vi "CreateExportedFunctionVIs.vi"   [LabVIEW 2020]
uses:
  <vilib>/Utility/traverseref.llb/TRef TravTarget.ctl
  6dd5ec1a-3140-4c59-8976-e265b4825e4e.vi
  c28e3e03-bc47-4083-b8a7-f1b137712541.vi
  82b46e61-a036-43bd-a8d9-afcc1ab177d3.vi
  337b4f8b-581d-4fd9-b696-00d79b3d5e3a.vi
  67cb83f1-d3a9-42e9-95c3-879ee97d33c6.vi
  533b81a4-3358-4744-80f6-d38457af82e6.vi
  g_industrial_cam/Camera/Get Pixel Format.vi
  g_industrial_cam/Camera/Set Pixel Format.vi
  g_industrial_cam/Camera/Get Exposure Time Bounds.vi
  g_industrial_cam/Camera/Available Pixel Formats.vi
  g_industrial_cam/Camera/Is Gain Available.vi
  g_industrial_cam/Camera/Get Height Increment.vi
  <vilib>/Comparison/Equal/Equal Functor/Equal Functor.lvclass
  <vilib>/Utility/traverseref.llb/VI Scripting - Traverse.lvlib
  g_industrial_cam/Camera/Camera.lvclass
types:
  T1 = typedef "TRef TravTarget.ctl" = enum16{"FP", "BD", "Other"}
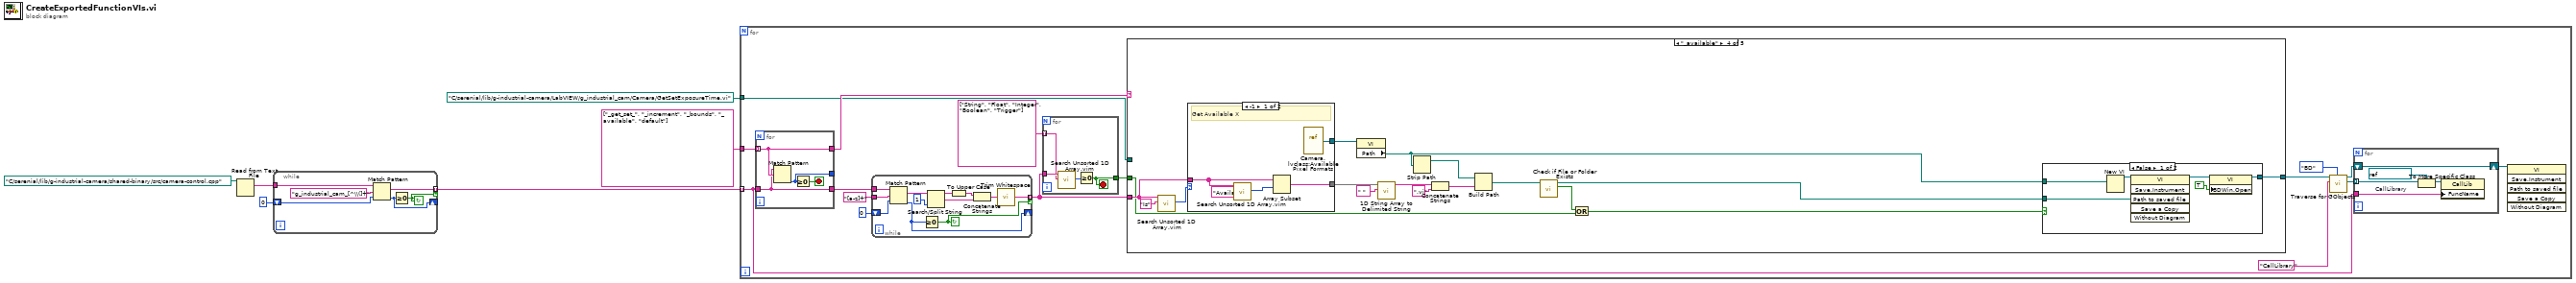
[diagram p0: block diagram]
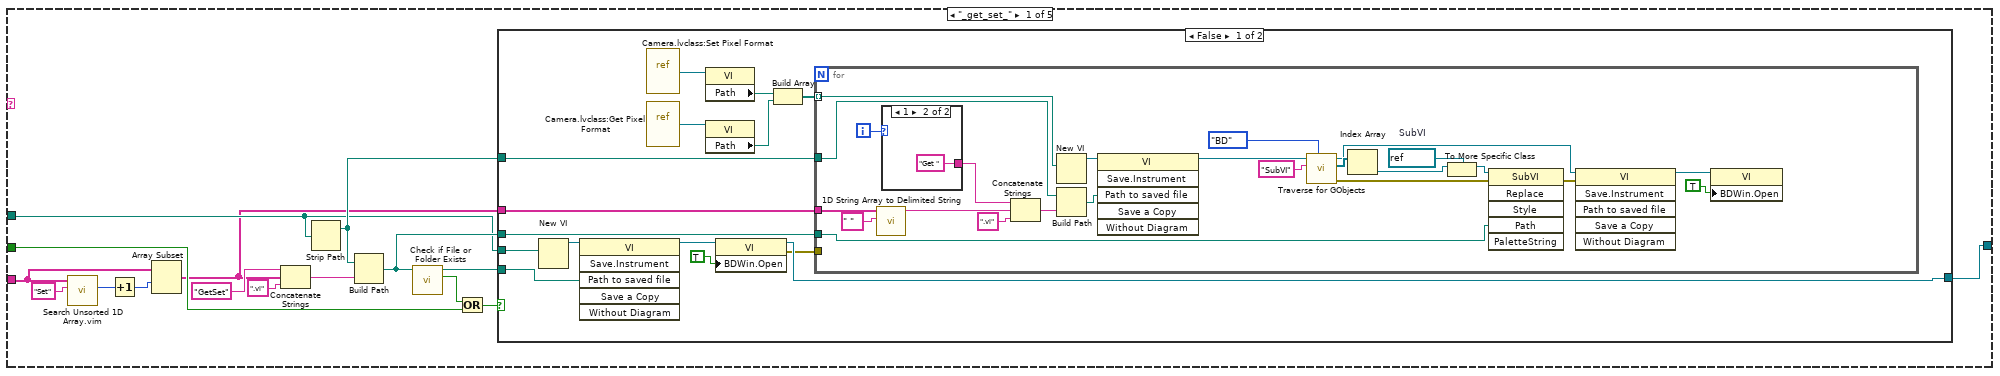
[diagram p2: hidden frame]
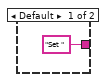
[diagram p3: hidden frame]
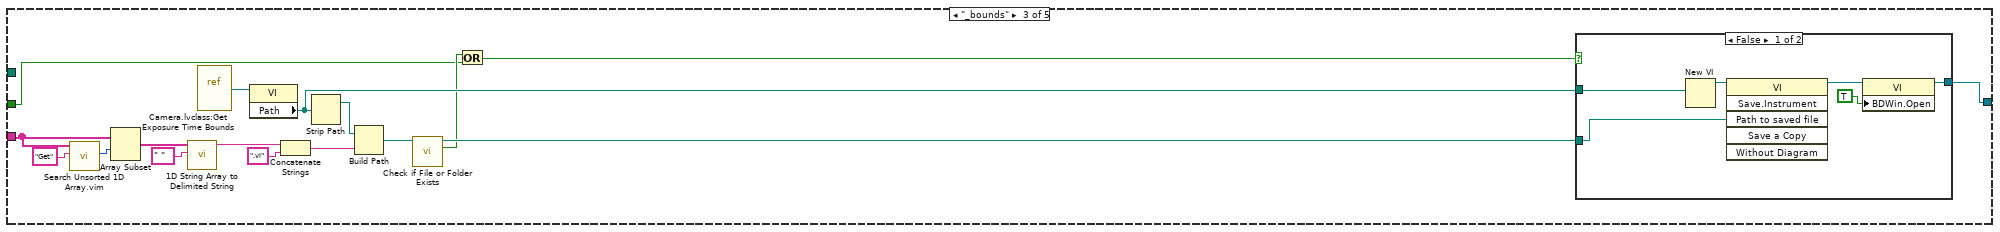
[diagram p6: hidden frame]
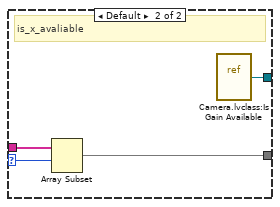
[diagram p8: hidden frame]
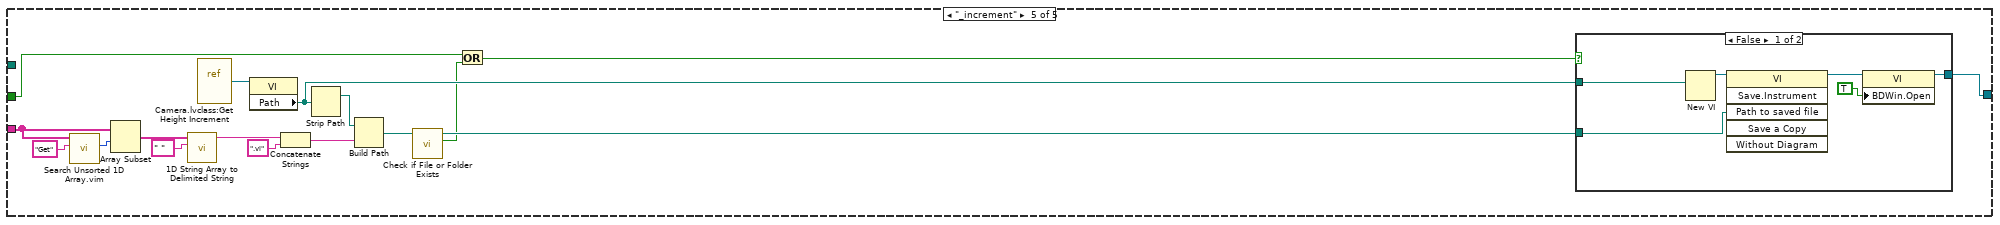
[diagram p10: hidden frame]
diagram:
  n1 = Read from Text File(file (use dialog)=path "C:/serenial/lib/g-industrial-camera/shared-binary/src/camera-control.cpp") -> (text=w1:string)  [unwired: 3 in, 3 out]
  n2 = while {
    tunnel: w1 -> [w12]
    shift-right: [w8] -> _
    shift-left: 0 ("offset (0)") -> [w10]
    tunnel: [w9] -> w5 mode=indexing if=w7
    stop <- w7 continue-if-true
    n3 = Match Pattern(string=w12, regular expression="g_industrial_cam_[^\\(]+", offset (0)=w10) -> (match substring=w9:string, offset past match=w8:i32)  [unwired: 2 out]
    n4 = Greater Or Equal To 0?(x=w8) -> (x >= 0?=w7:bool)
  }
  n5 = for {
    tunnel: w5 -> [w17] mode=indexing
    tunnel: string[] ["_get_set_", "_increment", "_bounds", "_available", "default"] -> [w28]
    tunnel: path "C:/serenial/lib/g-industrial-camera/LabVIEW/g_industrial_cam/Camera/GetSetExposureTime.vi" ("template") -> [w16]
    n6 = for {
      tunnel: w17 -> [w186]
      tunnel: w28 -> [w187] mode=indexing
      tunnel: [w187] -> w27
      tunnel: [w186] -> w26
      tunnel: [w185] -> _
      stop <- w188 stop-if-true
      n7 = Match Pattern(string=w186, regular expression=w187) -> (offset past match=w185:i32)  [unwired: 1 in, 3 out]
      n8 = Greater Or Equal To 0?(x=w185) -> (x >= 0?=w188:bool)
    }
    n9 = while {
      tunnel: w26 -> [w49]
      tunnel: "[a-z]+" ("regular expression") -> [w48]
      shift-right: [w46] -> _
      shift-left: 0 ("offset (0)") -> [w47]
      tunnel: [w38] -> w14 mode=indexing if=w45
      stop <- w45 continue-if-true
      n10 = Match Pattern(string=w49, regular expression=w48, offset (0)=w47) -> (match substring=w43:string, offset past match=w46:i32)  [unwired: 2 out]
      n11 = Greater Or Equal To 0?(x=w46) -> (x >= 0?=w45:bool)
      n12 = Search/Split String(string=w43, offset (0)=1) -> (substring before match=w42:string, match + rest of string=w40:string)  [unwired: 1 in, 1 out]
      n13 = To Upper Case(1:w42) -> (0:w41:string)
      n14 = Concatenate Strings(w41, w40) -> (w39:string)
      n15 = call <vilib>:"Trim Whitespace.vi"("string"=w39) -> ("trimmed string"=w38:string)  [unwired: 1 in]
    }
    n16 = for {
      tunnel: string[] ["String", "Float", "Integer", "Boolean", "Trigger"] -> [w31] mode=indexing
      tunnel: w14 -> [w32]
      tunnel: [w29] -> w13
      stop <- w29 stop-if-true
      n17 = call "Search Unsorted 1D Array.vim"("element"=w31, "unsorted 1D array"=w32) -> ("index of element"=w30:i32)  [unwired: 9 in]
      n18 = Greater Or Equal To 0?(x=w30) -> (x >= 0?=w29:bool)
    }
    n19 = case shown="\"_available\"" w27 {
      tunnel: w14 -> [w57 _ w122 w145 w177]
      tunnel: [w63 _ w111 w134 w166] -> w20
      tunnel: w16 -> [w55 _ _ _ _]
      tunnel: w13 -> [w51 _ w107 w130 w162]
      frame "_get_set_" {
        n20 = call "Search Unsorted 1D Array.vim"("element"="Set", "unsorted 1D array"=w57) -> ("index of element"=w58:i32)  [unwired: 9 in]
        n21 = Increment(x=w58) -> (x+1=w56:i32)
        n22 = Array Subset(array=w57, index=w56) -> (w50:string[])  [unwired: 1 in]
        n23 = Concatenate Strings("GetSet" ("string"), w50, ".vi" ("string")) -> (w64:string)
        n24 = Strip Path(path=w55) -> (stripped path=w62:path)  [unwired: 1 out]
        n25 = Build Path(base path=w62, name or relative path=w64) -> (appended path=w61:path)
        n26 = call <vilib>:"Check if File or Folder Exists.vi"("path"=w61) -> ("file or folder exists?"=w53:bool, "dup path"=w54:path)  [unwired: 8 in, 1 out]
        n27 = Or(x=w53, y=w51) -> (x .or. y?=w52:bool)
        n28 = case shown="False" w52 {
          tunnel: [w80 _] -> w63
          tunnel: w62 -> [w74 _]
          tunnel: w61 -> [w73 _]
          tunnel: w50 -> [w68 _]
          tunnel: w55 -> [w67 _]
          tunnel: w54 -> [w66 _]
          frame False {
            n29 = New VI(10:w67) -> (3:w71:refnum<vi>)  [unwired: 6 in, 1 out]
            n30 = invoke class="VI" method="Save.Instrument"(reference=w71, "Path to saved file"=w66) -> (reference out=w70:refnum<vi>)  [unwired: 4 in, 5 out]
            n31 = vi-ref "Camera.lvclass:Set Pixel Format.vi"() -> (w78:refnum<vi>)
            n32 = vi-ref "Camera.lvclass:Get Pixel Format.vi"() -> (w79:refnum<vi>)
            n33 = property class="VI"(reference=w78) -> ("Path"=w76:path)  [unwired: 1 in, 2 out]
            n34 = property class="VI"(reference=w79) -> ("Path"=w77:path)  [unwired: 1 in, 2 out]
            n35 = property class="VI"(reference=w70, "BDWin.Open"=TRUE ("Block Diagram Window:Open")) -> (reference out=w80:refnum<vi>, error out=w72:errorcluster)  [unwired: 1 in]
            n36 = Build Array(w76, w77) -> (w75:path[])
            n37 = for {
              tunnel: w75 -> [w99] mode=indexing
              tunnel: w74 -> [w100]
              tunnel: w68 -> [w97]
              tunnel: w73 -> [w98]
              tunnel: w72 -> [_]
              i -> [w96]
              w87 = refnum<vi> refnum  # SubVI
              n38 = call <vilib>:"1D String Array to Delimited String.vi"("delimiter"=" ", "string array"=w97) -> ("delimited string"=w103:string)  [unwired: 9 in]
              n39 = case shown="1" w96 {
                tunnel: ["Set " "Get "] -> w95
                frame Default {
                }
                frame 1 {
                }
              }
              n40 = Concatenate Strings(w95, w103, ".vi" ("string")) -> (w101:string)
              n41 = New VI(10:w99) -> (3:w94:refnum<vi>)  [unwired: 6 in, 1 out]
              n42 = Build Path(base path=w100, name or relative path=w101) -> (appended path=w93:path)
              n43 = invoke class="VI" method="Save.Instrument"(reference=w94, "Path to saved file"=w93) -> (reference out=w92:refnum<vi>)  [unwired: 4 in, 5 out]
              n44 = call <vilib>:"Traverse for GObjects.vi"("Traverse Target"=TRef_TravTarget."BD", "Class Name"="SubVI", "VI Refnum"=w92) -> ("error out"=w85:errorcluster, "References"=w89:refnum<vi>[], "dup VI Refnum"=w84:refnum<vi>)  [unwired: 5 in, 1 out]
              n45 = Index Array(array=w89) -> (element=w88:refnum<vi>)  [unwired: 1 in]
              n46 = To More Specific Class(target class=w87, reference=w88) -> (specific class reference=w86:refnum<vi>)  [unwired: 1 in, 1 out]
              n47 = invoke class="SubVI" method="Replace"(reference=w86, error in=w85, "Path"=w98) -> (error out=w83:errorcluster)  [unwired: 3 in, 5 out]
              n48 = invoke class="VI" method="Save.Instrument"(reference=w84, error in=w83) -> (reference out=w82:refnum<vi>)  [unwired: 4 in, 5 out]
              n49 = property class="VI"(reference=w82, "BDWin.Open"=TRUE ("Block Diagram Window:Open")) -> ()  [unwired: 1 in, 2 out]
            }
          }
          frame True {
          }
        }
      }
      frame Default {
      }
      frame "_bounds" {
        n50 = call "Search Unsorted 1D Array.vim"("element"="Get", "unsorted 1D array"=w122) -> ("index of element"=w121:i32)  [unwired: 9 in]
        n51 = Array Subset(array=w122, index=w121) -> (w118:string[])  [unwired: 1 in]
        n52 = call <vilib>:"1D String Array to Delimited String.vi"("delimiter"=" ", "string array"=w118) -> ("delimited string"=w116:string)  [unwired: 9 in]
        n53 = vi-ref "Camera.lvclass:Get Exposure Time Bounds.vi"() -> (w120:refnum<vi>)
        n54 = property class="VI"(reference=w120) -> ("Path"=w115:path)  [unwired: 1 in, 2 out]
        n55 = Concatenate Strings(w116, ".vi" ("string")) -> (w113:string)
        n56 = Strip Path(path=w115) -> (stripped path=w114:path)  [unwired: 1 out]
        n57 = Build Path(base path=w114, name or relative path=w113) -> (appended path=w112:path)
        n58 = call <vilib>:"Check if File or Folder Exists.vi"("path"=w112) -> ("file or folder exists?"=w109:bool, "dup path"=w110:path)  [unwired: 8 in, 1 out]
        n59 = Or(x=w109, y=w107) -> (x .or. y?=w108:bool)
        n60 = case shown="False" w108 {
          tunnel: w115 -> [w128 _]
          tunnel: [w125 _] -> w111
          tunnel: w110 -> [w124 _]
          frame False {
            n61 = New VI(10:w128) -> (3:w129:refnum<vi>)  [unwired: 6 in, 1 out]
            n62 = invoke class="VI" method="Save.Instrument"(reference=w129, "Path to saved file"=w124) -> (reference out=w127:refnum<vi>)  [unwired: 4 in, 5 out]
            n63 = property class="VI"(reference=w127, "BDWin.Open"=TRUE ("Block Diagram Window:Open")) -> (reference out=w125:refnum<vi>)  [unwired: 1 in, 1 out]
          }
          frame True {
          }
        }
      }
      frame "_available" {
        n64 = call "Search Unsorted 1D Array.vim"("element"="Is", "unsorted 1D array"=w145) -> ("index of element"=w144:i32)  [unwired: 9 in]
        n65 = case shown="-1" w144 {
          selector: w144 -> [_ w154]
          tunnel: w145 -> [w150 w155]
          tunnel: [w147 w153] -> w143
          tunnel: [w148 w152] -> w141
          frame -1 {
            # "Get Available X"
            n66 = call "Search Unsorted 1D Array.vim"("element"="Available", "unsorted 1D array"=w150) -> ("index of element"=w149:i32)  [unwired: 9 in]
            n67 = Array Subset(array=w150, index=w149) -> (w148:string[])  [unwired: 1 in]
            n68 = vi-ref "Camera.lvclass:Available Pixel Formats.vi"() -> (w147:refnum<vi>)
          }
          frame Default {
            # "is_x_avaliable"
            n69 = Array Subset(array=w155, index=w154) -> (w152:string[])  [unwired: 1 in]
            n70 = vi-ref "Camera.lvclass:Is Gain Available.vi"() -> (w153:refnum<vi>)
          }
        }
        n71 = property class="VI"(reference=w143) -> ("Path"=w138:path)  [unwired: 1 in, 2 out]
        n72 = call <vilib>:"1D String Array to Delimited String.vi"("delimiter"=" ", "string array"=w141) -> ("delimited string"=w139:string)  [unwired: 9 in]
        n73 = Strip Path(path=w138) -> (stripped path=w137:path)  [unwired: 1 out]
        n74 = Concatenate Strings(w139, ".vi" ("string")) -> (w136:string)
        n75 = Build Path(base path=w137, name or relative path=w136) -> (appended path=w135:path)
        n76 = call <vilib>:"Check if File or Folder Exists.vi"("path"=w135) -> ("file or folder exists?"=w132:bool, "dup path"=w133:path)  [unwired: 8 in, 1 out]
        n77 = Or(x=w132, y=w130) -> (x .or. y?=w131:bool)
        n78 = case shown="False" w131 {
          tunnel: w138 -> [w160 _]
          tunnel: [w157 _] -> w134
          tunnel: w133 -> [w156 _]
          frame False {
            n79 = New VI(10:w160) -> (3:w161:refnum<vi>)  [unwired: 6 in, 1 out]
            n80 = invoke class="VI" method="Save.Instrument"(reference=w161, "Path to saved file"=w156) -> (reference out=w159:refnum<vi>)  [unwired: 4 in, 5 out]
            n81 = property class="VI"(reference=w159, "BDWin.Open"=TRUE ("Block Diagram Window:Open")) -> (reference out=w157:refnum<vi>)  [unwired: 1 in, 1 out]
          }
          frame True {
          }
        }
      }
      frame "_increment" {
        n82 = call "Search Unsorted 1D Array.vim"("element"="Get", "unsorted 1D array"=w177) -> ("index of element"=w176:i32)  [unwired: 9 in]
        n83 = Array Subset(array=w177, index=w176) -> (w173:string[])  [unwired: 1 in]
        n84 = call <vilib>:"1D String Array to Delimited String.vi"("delimiter"=" ", "string array"=w173) -> ("delimited string"=w171:string)  [unwired: 9 in]
        n85 = vi-ref "Camera.lvclass:Get Height Increment.vi"() -> (w175:refnum<vi>)
        n86 = property class="VI"(reference=w175) -> ("Path"=w170:path)  [unwired: 1 in, 2 out]
        n87 = Concatenate Strings(w171, ".vi" ("string")) -> (w168:string)
        n88 = Strip Path(path=w170) -> (stripped path=w169:path)  [unwired: 1 out]
        n89 = Build Path(base path=w169, name or relative path=w168) -> (appended path=w167:path)
        n90 = call <vilib>:"Check if File or Folder Exists.vi"("path"=w167) -> ("file or folder exists?"=w164:bool, "dup path"=w165:path)  [unwired: 8 in, 1 out]
        n91 = Or(x=w162, y=w164) -> (x .or. y?=w163:bool)
        n92 = case shown="False" w163 {
          tunnel: w170 -> [w183 _]
          tunnel: [w180 _] -> w166
          tunnel: w165 -> [w179 _]
          frame False {
            n93 = New VI(10:w183) -> (3:w184:refnum<vi>)  [unwired: 6 in, 1 out]
            n94 = invoke class="VI" method="Save.Instrument"(reference=w184, "Path to saved file"=w179) -> (reference out=w182:refnum<vi>)  [unwired: 4 in, 5 out]
            n95 = property class="VI"(reference=w182, "BDWin.Open"=TRUE ("Block Diagram Window:Open")) -> (reference out=w180:refnum<vi>)  [unwired: 1 in, 1 out]
          }
          frame True {
          }
        }
      }
    }
    n96 = call <vilib>:"Traverse for GObjects.vi"("Traverse Target"=TRef_TravTarget."BD", "Class Name"="CallLibrary", "VI Refnum"=w20) -> ("References"=w21:refnum<vi>[], "dup VI Refnum"=w19:refnum<vi>)  [unwired: 5 in, 2 out]
    n97 = for {
      tunnel: w21 -> [w36] mode=indexing
      tunnel: w17 -> [w34]
      shift-right: [w33] -> w18
      shift-left: w19 -> [w33]
      w37 = refnum<vi> refnum  # CallLibrary
      n98 = To More Specific Class(target class=w37, reference=w36) -> (specific class reference=w35:refnum<vi>)  [unwired: 1 in, 1 out]
      n99 = property class="CallLib"(reference=w35, "FuncName"=w34) -> ()  [unwired: 1 in, 2 out]
    }
    n100 = invoke class="VI" method="Save.Instrument"(reference=w18) -> ()  [unwired: 5 in, 6 out]
  }
